vi "Write configuration.vi"(8 "error in":errorcluster, 10 "configuration":refnum<class "NISE_CEF_serializable configuration.lvclass">, 11 "CVT editor node in":refnum<class "CVT editor node.lvclass">) -> (0 "error out":errorcluster, 3 "CVT editor node out":refnum<class "CVT editor node.lvclass">)   [LabVIEW 2013, in "CVT editor node.lvclass"]
uses:
  CVT editor node.lvclass
  <vilib>/NI/Configuration Framework/serializable configuration/NISE_CEF_serializable configuration.lvclass
  configuration/CVT configuration.lvclass
  CVT editor node.lvclass/CVT editor node.ctl
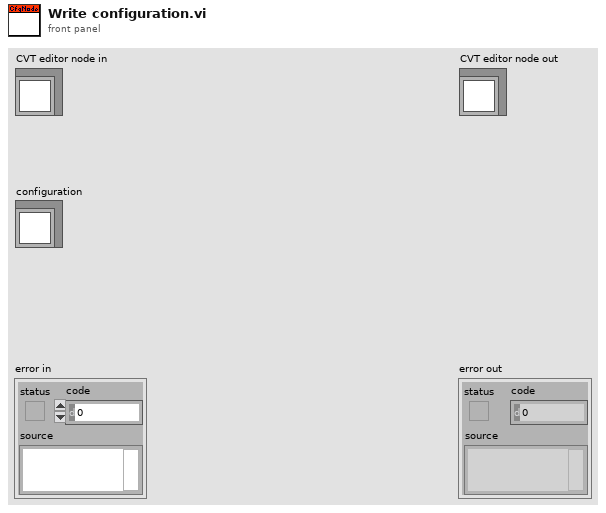
[diagram p1: front panel]
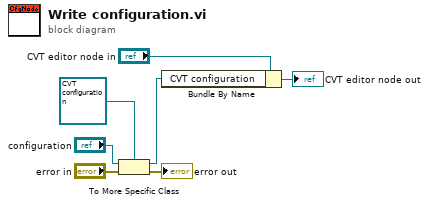
[diagram p0: block diagram]
diagram:
  n1 = To More Specific Class(target class=refnum<class "CVT configuration.lvclass"> refnum ("CVT configuration"), reference="configuration", error in="error in") -> (specific class reference=w1:refnum<class "CVT configuration.lvclass">, error out=→"error out":errorcluster)
  n2 = Bundle By Name(cluster="CVT editor node in", "CVT configuration"=w1) -> (→"CVT editor node out":refnum<class "CVT editor node.lvclass">)
